vi "Custom Error Message 2012 NIVerified.vi"() -> ()   [LabVIEW 2012]
doc: "This VI demonstrates how to generate a custom error message in LabVIEW."
panel:
  in  "Use Custom Message?":bool
  out "Original Error Cluster":errorcluster
  # "Overview: Demonstrates how to generate a custom error message in LabVIEW. \nRequirements:  LabVIEW 2012 (or compatible)  \nInstructions:\n1. Define your preferred value for the \"Use Custom Message?\" boolean.\n2. Enter your preferred error message.\n3. Run the VI."
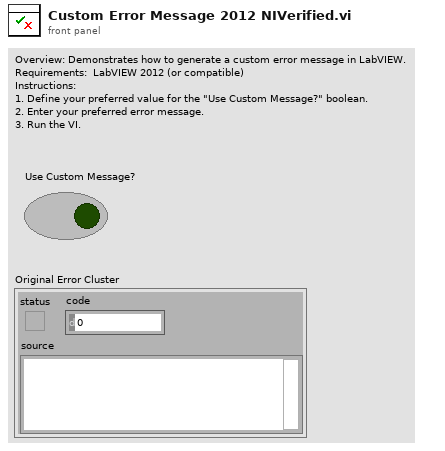
[diagram p1: front panel]
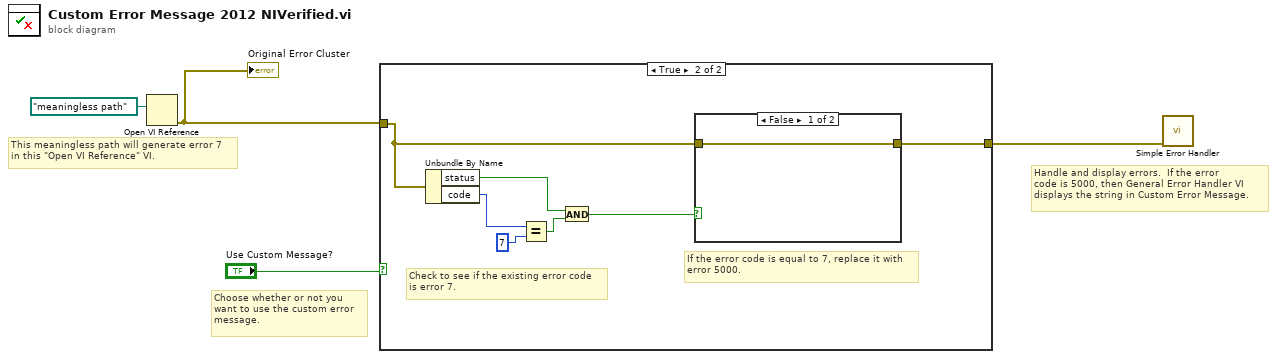
[diagram p0: block diagram]
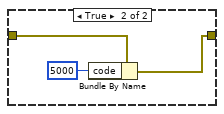
[diagram p3: hidden frame]
diagram:
  # "Handle and display errors.  If the error\ncode is 5000, then General Error Handler VI\ndisplays the string in Custom Error Message."
  # "Choose whether or not you\nwant to use the custom error\nmessage."
  # "This meaningless path will generate error 7\nin this \"Open VI Reference\" VI."
  n1 = Open VI Reference(vi path=path "meaningless path") -> (error out=w1:errorcluster)  [unwired: 5 in, 1 out]
  "Original Error Cluster" <- w1
  n2 = case shown="True" "Use Custom Message?" {
    tunnel: w1 -> [w5 w7]
    tunnel: [w5 w6] -> w2
    frame False {
    }
    frame True {
      # "If the error code is equal to 7, replace it with\nerror 5000."
      # "Check to see if the existing error code\nis error 7."
      n3 = Unbundle By Name(w7) -> ("status"=w12:bool, "code"=w9:i32)
      n4 = Equal?(x=w9, y=7) -> (x = y?=w11:bool)
      n5 = And(x=w12, y=w11) -> (x .and. y?=w8:bool)
      n6 = case shown="False" w8 {
        tunnel: w7 -> [w13 w14]
        tunnel: [w13 w15] -> w6
        frame False {
        }
        frame True {
          n7 = Bundle By Name(cluster=w14, "code"=5000) -> (w15:errorcluster)
        }
      }
    }
  }
  n8 = call <vilib>:"Simple Error Handler.vi"("error in (no error)"=w2) -> ()  [unwired: 4 in, 5 out]
